vi "extract fit locations to readings.vi"(6 "tmin":dbl, 7 "tmax":dbl, 8 "error in (no error)":errorcluster, 11 "fitLocation queue":refnum<queue>) -> (0 "error out":errorcluster, 3 "positions as reading array":T1[](array[typedef]))   [LabVIEW 2017]
uses:
  typedefs/magnet location with timestamp.ctl
  typedefs/reading.ctl
  typedefs/readingType.ctl
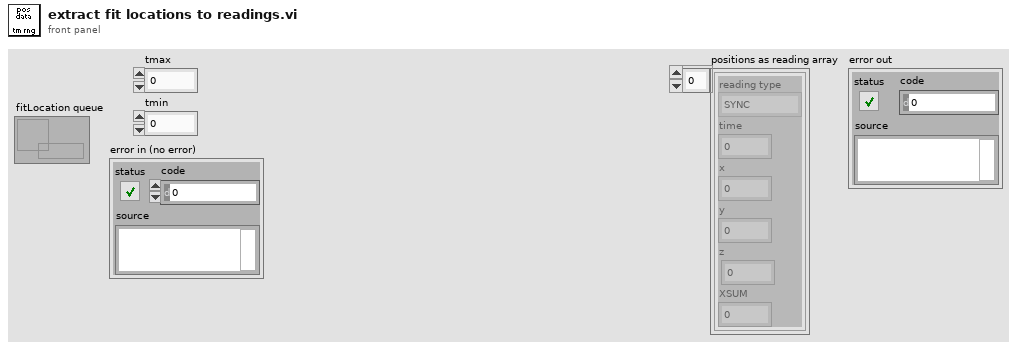
[diagram p1: front panel]
types:
  T1 = typedef "reading.ctl" = cluster{"reading type":T2, "time":fxp<+,48,48>, "x":sgl, "y":sgl, "z":sgl, "XSUM":u8}
  T2 = typedef "readingType.ctl" = enum8{"SYNC", "DETVAL", "COILI", "MAGVEC", "ACCVEC", "CROSSING", "MAGVEC0", "MAGVEC1", "MAGVEC2", "MAGVEC3", "MAGVEC4", "MAGVEC5", "MAGVEC6", "MAGVEC7"}
  T3 = typedef "magnet location with timestamp.ctl" = cluster{"x magnet":dbl, "y magnet":dbl, "z magnet":dbl, "Br*V (T*mm^3)":dbl, "theta - moment angle to z-axis":dbl, "phi - moment angle to x-axis":dbl, "measurement time":dbl}
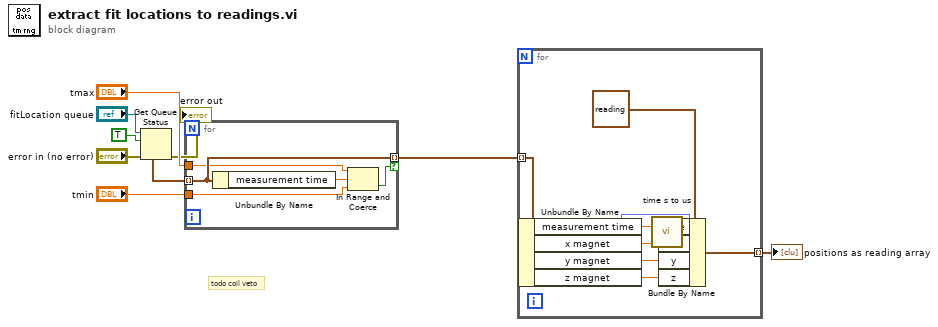
[diagram p0: block diagram]
diagram:
  # "todo coil veto"
  n1 = Get Queue Status(queue="fitLocation queue", return elements? (F)=TRUE, error in (no error)="error in (no error)") -> (error out=→"error out":errorcluster, elements=w7:T3[])  [unwired: 6 out]
  n2 = for {
    tunnel: w7 -> [w14] mode=indexing
    tunnel: [w14] -> w3 mode=indexing if=w12
    tunnel: "tmax" -> [w11]
    tunnel: "tmin" -> [w10]
    n3 = Unbundle By Name(w14) -> ("measurement time"=w13:dbl)
    n4 = In Range and Coerce(upper limit=w11, x=w13, lower limit=w10) -> (In Range?=w12:bool)  [unwired: 1 out]
  }
  n5 = for {
    tunnel: w3 -> [w21] mode=indexing
    tunnel: [w15] -> w2 mode=indexing
    n6 = Unbundle By Name(w21) -> ("measurement time"=w20:dbl, "x magnet"=w18:dbl, "y magnet"=w17:dbl, "z magnet"=w16:dbl)
    n7 = call "time s to us.vi"("time (s)"=w20) -> ("time (us)"=w19:fxp<+,48,48>)  [unwired: 10 in]
    n8 = Bundle By Name(cluster=T1 {"reading type"=enum."SYNC", "time"=0.0, "x"=0.0, "y"=0.0, "z"=0.0, "XSUM"=0} ("reading"), "time"=w19, "x"=w18, "y"=w17, "z"=w16) -> (w15:T1)
  }
  "positions as reading array" <- w2
